vi "Fetch (Multiple) Binary.vi"(0 "VISA resource name":refnum<visa-resource-name>, 1 "Start Index (1)":i32=1, 2 "Buffer Elements 1":u16(ring) items=["Date", "Extra", "Formatted", "Fractional", "Relative", "Seconds", "Status", "Time", "Timestamp", "Unit", "Reading"], 5 "Buffer Name ()":string, 7 "Data Format":u16(ring) items=["Single precision", "Double precision"], 9 "Timeout (100000 ms)":i32=100000, 11 "error in (no error)":errorcluster, 12 "End Index (10)":i32=10, 13 "Buffer Elements  2":u16(ring) items=["Date", "Extra", "Formatted", "Fractional", "Relative", "Seconds", "Status", "Time", "Timestamp", "Unit", "Reading"]) -> (4 "VISA resource name out":refnum<visa-resource-name>, 6 "Measurements":dbl[](array[numeric]), 15 "error out":errorcluster)   [LabVIEW 2021, in "Keithley DMM7510.lvlib"]
doc: "Reads and returns multiple measurements from the instrument. The data are extracted in binary format then converted to Single format measurements. Use this VI when you want to take multiple measurements using an immediate trigger. Use the low-level VIs for other triggering options."
uses:
  Keithley DMM7510.lvlib
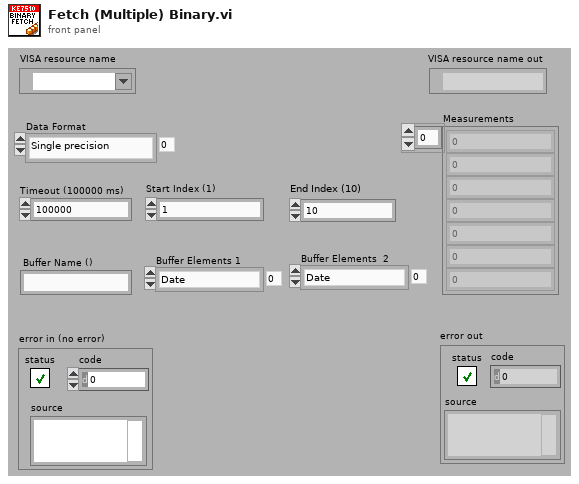
[diagram p1: front panel]
types:
  T1 = enum16{"big-endian, network order", "native, host order", "little-endian"}
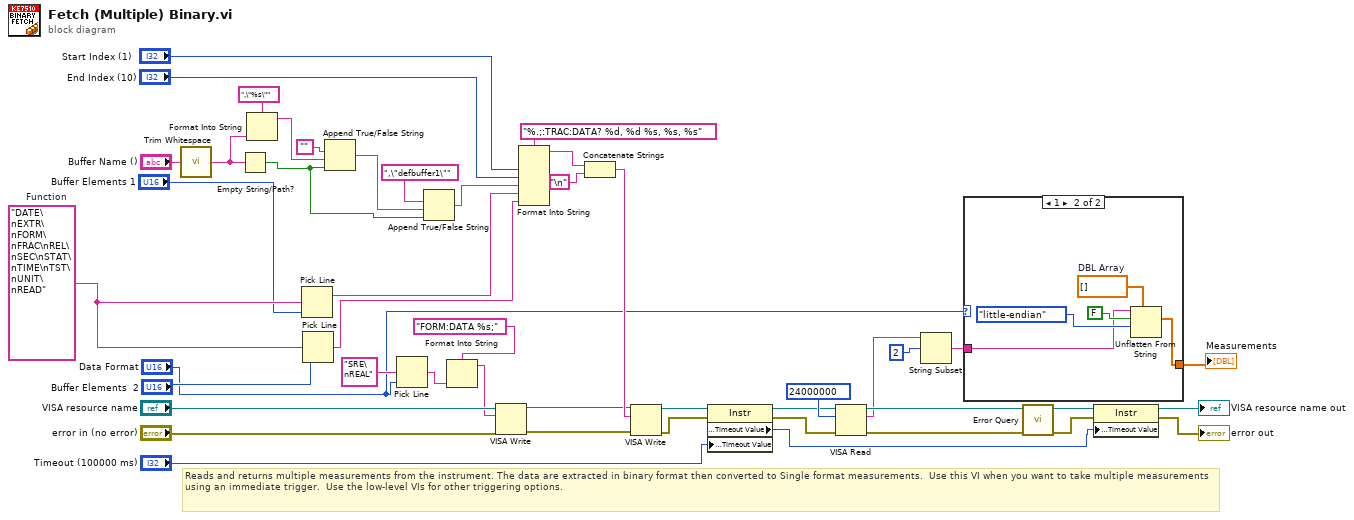
[diagram p0: block diagram]
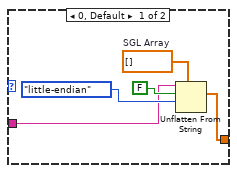
[diagram p2: hidden frame]
diagram:
  w11 = "DATE\nEXTR\nFORM\nFRAC\nREL\nSEC\nSTAT\nTIME\nTST\nUNIT\nREAD"  # Function
  # "Reads and returns multiple measurements from the instrument. The data are extracted in binary format then converted to Single format measurements.  Use this VI when you want to take multiple measurements using an immediate trigger.  Use the low-level VIs for other triggering options."
  n1 = call <vilib>:"Trim Whitespace.vi"("string"="Buffer Name ()") -> ("trimmed string"=w19:string)  [unwired: 1 in]
  n2 = Empty String/Path?(string/path=w19) -> (empty?=w1:bool)
  n3 = Format Into String(format string=",\"%s\"", w19) -> (resulting string=w40:string)  [unwired: 2 in, 1 out]
  n4 = Pick Line(multi-line string=w11, line index="Buffer Elements 1") -> (output string=w24:string)  [unwired: 1 in]
  n5 = Pick Line(multi-line string=w11, line index="Buffer Elements  2") -> (output string=w23:string)  [unwired: 1 in]
  n6 = Append True/False String(1:w1, 2:w40, 3:"") -> (0:w21:string)  [unwired: 1 in]
  n7 = Pick Line(multi-line string="SRE\nREAL", line index="Data Format") -> (output string=w4:string)  [unwired: 1 in]
  n8 = Append True/False String(1:w1, 2:w21, 3:",\"defbuffer1\"" ("true string")) -> (0:w22:string)  [unwired: 1 in]
  n9 = Format Into String(format string="FORM:DATA %s;", w4) -> (resulting string=w3:string)  [unwired: 2 in, 1 out]
  n10 = VISA Write(VISA resource name="VISA resource name", write buffer=w3, error in (no error)="error in (no error)") -> (VISA resource name out=w7:refnum<visa-resource-name>, error out=w8:errorcluster)  [unwired: 1 out]
  n11 = Format Into String(format string="%.;:TRAC:DATA? %d, %d %s, %s, %s", "Start Index (1)", "End Index (10)", w22, w24, w23) -> (resulting string=w28:string)  [unwired: 2 in, 1 out]
  n12 = Concatenate Strings(w28, "\n") -> (w43:string)
  n13 = VISA Write(VISA resource name=w7, write buffer=w43, error in (no error)=w8) -> (VISA resource name out=w38:refnum<visa-resource-name>, error out=w37:errorcluster)  [unwired: 1 out]
  n14 = property on="Property Node" class="Instr"(reference=w38, error in=w37, "General Settings:Timeout Value"="Timeout (100000 ms)") -> (reference out=w35:refnum<visa-resource-name>, error out=w36:errorcluster, "General Settings:Timeout Value"=w30:u32)
  n15 = VISA Read(VISA resource name=w35, byte count=i64 24000000, error in (no error)=w36) -> (VISA resource name out=w45:refnum<visa-resource-name>, read buffer=w15:string, error out=w44:errorcluster)  [unwired: 1 out]
  n16 = String Subset(string=w15, offset (0)=2) -> (substring=w16:string)  [unwired: 1 in]
  n17 = case shown="1" "Data Format" {
    tunnel: [w48 w53] -> w17
    tunnel: w16 -> [w47 w52]
    frame 0, Default {
      w51 = sgl[] []  # SGL Array
      n18 = Unflatten From String(type=w51, binary string=w47, data includes array or string size? (T)=FALSE, byte order (0:big-endian, network order)=T1."little-endian") -> (value=w48:sgl[])  [unwired: 1 in, 2 out]
    }
    frame 1 {
      w56 = dbl[] []  # DBL Array
      n19 = Unflatten From String(type=w56, binary string=w52, data includes array or string size? (T)=FALSE, byte order (0:big-endian, network order)=T1."little-endian") -> (value=w53:dbl[])  [unwired: 1 in, 2 out]
    }
  }
  "Measurements" <- w17
  n20 = call "Error Query.vi"("error in (no error)"=w44, "VISA resource name"=w45) -> ("error out"=w32:errorcluster, "VISA resource name out"=w34:refnum<visa-resource-name>)  [unwired: 6 in, 2 out]
  n21 = property on="Property Node" class="Instr"(reference=w34, error in=w32, "General Settings:Timeout Value"=w30) -> (reference out=→"VISA resource name out":refnum<visa-resource-name>, error out=→"error out":errorcluster)
